vi "FlatToRichnise_ConnectInfo.vi"(5 "OutputClusterType":T1, 11 "InputCluster":T5) -> (3 "OutputCluster":T1)   [LabVIEW 2021, in "basic_switch_executive_driver_client.lvlib"]
uses:
  basic_switch_executive_driver_client.lvlib
  nise_ConnectInfo_Flat.ctl
  nise_SessionInformation_Flat.ctl
  nise_MulticonnectMode.ctl
  nise_ConnectInfo.ctl
  nise_SessionInformation.ctl
  <vilib>/Plug-In SDKs/Clients/Session Management V1/Session Reservation/Initialize and Close Session Behavior.ctl
  <vilib>/Plug-In SDKs/Clients/Session Management V1/Session Reservation/Session Reservation.lvclass
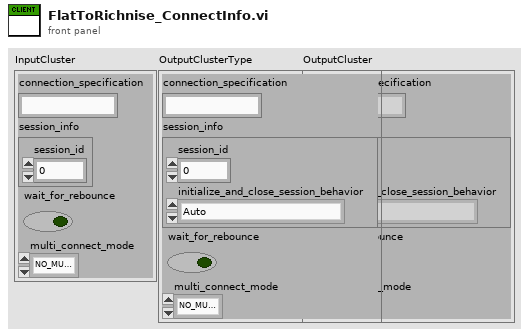
[diagram p1: front panel]
types:
  T1 = typedef "basic_switch_executive_driver_client.lvlib/nise_ConnectInfo.ctl" = cluster{"connection_specification":string, "session_info":T2, "wait_for_rebounce":bool, "multi_connect_mode":T4}
  T2 = typedef "basic_switch_executive_driver_client.lvlib/nise_SessionInformation.ctl" = cluster{"session_id":u32, "initialize_and_close_session_behavior":T3}
  T3 = typedef "NI Session Management V1 Client.lvlib/Session Reservation.lvclass/Initialize and Close Session Behavior.ctl" = enum16{"Auto", "Initialize and Close", "Attach and Detach", "Initialize and Detach", "Attach and Close"}
  T4 = typedef "basic_switch_executive_driver_client.lvlib/nise_MulticonnectMode.ctl" = enum32{"NO_MULTICONNECT", "USE_DEFAULT_MODE", "MULTICONNECT_ROUTES"}
  T5 = typedef "basic_switch_executive_driver_client.lvlib/nise_ConnectInfo_Flat.ctl" = cluster{"connection_specification":string, "session_info":T6, "wait_for_rebounce":bool, "multi_connect_mode":T4}
  T6 = typedef "basic_switch_executive_driver_client.lvlib/nise_SessionInformation_Flat.ctl" = cluster{"session_id":u32}
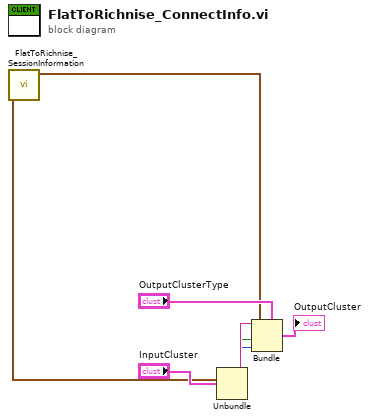
[diagram p0: block diagram]
diagram:
  n1 = Unbundle "Unbundle"("InputCluster") -> ("connection_specification"=w5:string, "session_info"=w4:T6, "wait_for_rebounce"=w2:bool, "multi_connect_mode"=w1:T4)
  n2 = call "FlatToRichnise_SessionInformation.vi"("InputCluster"=w4) -> ("OutputCluster"=w3:T2)  [unwired: 10 in]
  n3 = Bundle "Bundle"(cluster="OutputClusterType", "connection_specification"=w5, "session_info"=w3, "wait_for_rebounce"=w2, "multi_connect_mode"=w1) -> (→"OutputCluster":T1)
